vi "config CANcoder.vi"(8 "error in (no error)":errorcluster, 11 "CANcoder init data":T1={"description"="", "Installed?"=FALSE, "CAN ID"=0, "CAN Bus"="", "refnum name"="", "Sensor Direction"=FALSE, "Magnet Offset (Degrees)"=0.0, "gear ratio"=1.0} {"gear ratio" format="%_5f"}) -> (0 "error out":errorcluster)   [LabVIEW 2023]
uses:
  ctrl defs/ctrl CANcoder.ctl
  <vilib>/Rock Robotics/WPI/ThirdParty/Phoenix-LabVIEW/CANCoder/Controls/CTRE_Phoenix_CANcoder_Configurables.ctl
  <vilib>/Rock Robotics/WPI/ThirdParty/Phoenix-LabVIEW/CANCoder/Controls/CTRE_Phoenix_CANcoder_SensorInitializationStrategy.ctl
  <vilib>/Rock Robotics/WPI/ThirdParty/Phoenix-LabVIEW/CANCoder/Controls/CTRE_Phoenix_CANcoder_AbsoluteSensorRange.ctl
  <vilib>/Rock Robotics/WPI/ThirdParty/Phoenix-LabVIEW/Motor Controller/Controls/CTRE_Phoenix_MotorControl_VelocityMeasurementPeriod.ctl
  <vilib>/Rock Robotics/WPI/ThirdParty/Phoenix-LabVIEW/CANCoder/Controls/CTRE_Phoenix_CANcoder_SensorTimeBase.ctl
  <vilib>/Rock Robotics/WPI/ThirdParty/Phoenix-LabVIEW/CANCoder/Set/CTRE_Phoenix_CANcoder_SetPositionToAbsolute.vi
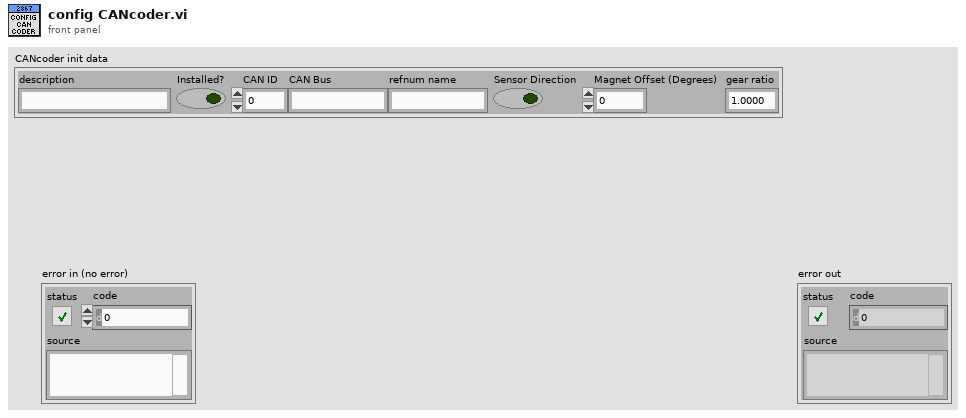
[diagram p1: front panel]
types:
  T1 = typedef "ctrl CANcoder.ctl" = cluster{"description":string, "Installed?":bool, "CAN ID":u8, "CAN Bus":string, "refnum name":string, "Sensor Direction":bool, "Magnet Offset (Degrees)":dbl, "gear ratio":dbl}
  T2 = typedef "CTRE_Phoenix_CANcoder_Configurables.ctl" = cluster{"Sensor Initialization Strategy":T3, "Absolute Sensor Range":T4, "Velocity Measurement Period":T5, "Velocity Measurement Window":i32, "Magnet Offset (Degrees)":dbl, "Sensor Direction":bool, "Sensor Coefficient":dbl, "Unit String":string, "Sensor Time Base":T6}
  T3 = typedef "CTRE_Phoenix_CANcoder_SensorInitializationStrategy.ctl" = enum16{"Boot To Zero", "Boot To Absolute Position"}
  T4 = typedef "CTRE_Phoenix_CANcoder_AbsoluteSensorRange.ctl" = enum16{"Unsigned [0 to 360)", "Signed [-180 to +180)"}
  T5 = typedef "CTRE_Phoenix_MotorControl_VelocityMeasurementPeriod.ctl" = u16
  T6 = typedef "CTRE_Phoenix_CANcoder_SensorTimeBase.ctl" = enum16{"Per100Ms_Legacy", "PerSecond", "PerMinute"}
  T7 = typedef "CTRE_Phoenix_CANcoder_DeviceRef.ctl" = cluster{"DeviceStatus":errorcluster, "Device Number":u8, "Handle":u64, "UsageFrame":u32, "Library Path":path}
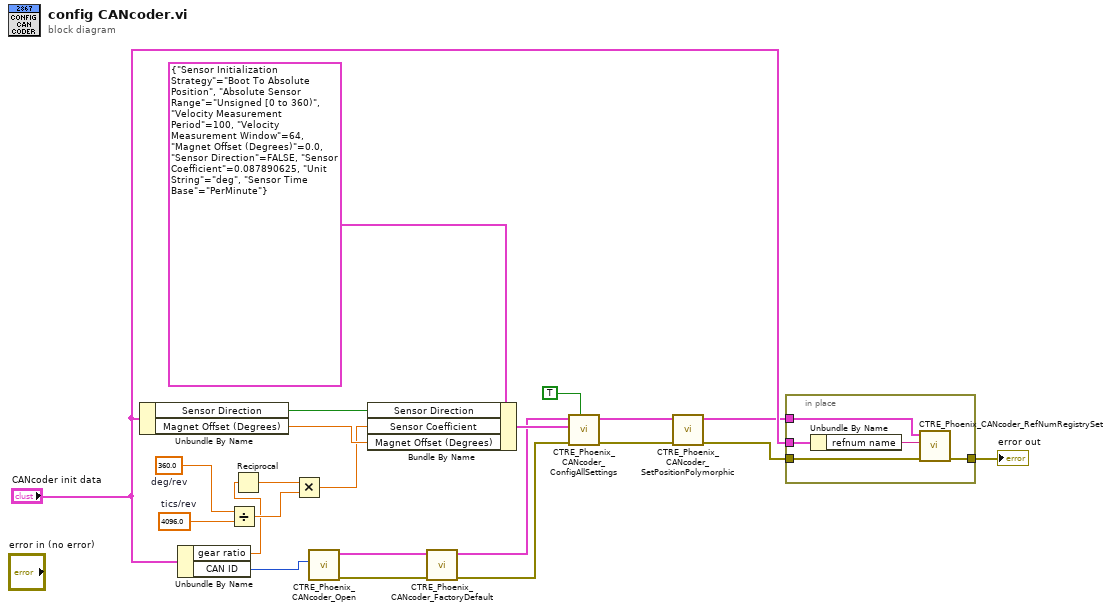
[diagram p0: block diagram]
diagram:
  w4 = 4096.0  # tics/rev
  w5 = 360.0  # deg/rev
  n1 = Unbundle By Name("CANcoder init data") -> ("Sensor Direction"=w14:bool, "Magnet Offset (Degrees)"=w13:dbl)
  n2 = Unbundle By Name("CANcoder init data") -> ("gear ratio"=w2:dbl, "CAN ID"=w21:u8)
  n3 = Divide(x=w5, y=w4) -> (x/y=w3:dbl)
  n4 = Reciprocal(x=w2) -> (1/x=w6:dbl)
  n5 = Multiply(x=w6, y=w3) -> (x*y=w1:dbl)
  n6 = call <vilib>:"CTRE_Phoenix_CANcoder_Open.vi"("Device Number"=w21) -> ("error out"=w20:errorcluster, "CTRE_CANcoder_DeviceRef"=w22:T7)  [unwired: 9 in]
  n7 = Bundle By Name(cluster=T2 {"Sensor Initialization Strategy"=enum."Boot To Absolute Position", "Absolute Sensor Range"=enum."Unsigned [0 to 360)", "Velocity Measurement Period"=100, "Velocity Measurement Window"=64, "Magnet Offset (Degrees)"=0.0, "Sensor Direction"=FALSE, "Sensor Coefficient"=0.087890625, "Unit String"="deg", "Sensor Time Base"=enum."PerMinute"} ("CANcoder Configurables"), "Sensor Direction"=w14, "Sensor Coefficient"=w1, "Magnet Offset (Degrees)"=w13) -> (w15:T2)
  n8 = call <vilib>:"CTRE_Phoenix_CANcoder_FactoryDefault.vi"("error in"=w20, "CTRE_CANcoder_DeviceRef"=w22) -> ("error out"=w11:errorcluster, "CTRE_CANcoder_DeviceRef"=w12:T7)  [unwired: 8 in]
  n9 = call <vilib>:"CTRE_Phoenix_CANcoder_ConfigAllSettings.vi"("Force Write"=TRUE, "error in (no error)"=w11, "CANcoder Configurables"=w15, "CTRE_CANcoder_DeviceRef"=w12) -> ("error out"=w9:errorcluster, "CTRE_CANcoder_DeviceRef"=w10:T7)  [unwired: 6 in]
  n10 = call-poly <vilib>:"CTRE_Phoenix_CANcoder_SetPositionPolymorphic.vi"("error in (no error)"=w9, "CTRE_CANcoder_DeviceRef"=w10) -> ("error out"=w7:errorcluster, "CTRE_CANcoder_DeviceRef"=w8:T7)  [unwired: 8 in]
  n11 = in-place {
    in-place-border: [w26] -> w19
    in-place-border: "CANcoder init data" -> [w25]
    in-place-border: w8 -> [w24]
    in-place-border: w7 -> [w23]
    n12 = Unbundle By Name(w25) -> ("refnum name"=w27:string)
    n13 = call <vilib>:"CTRE_Phoenix_CANcoder_RefNumRegistrySet.vi"("error in (no error)"=w23, "refnum name"=w27, "CTRE_CANcoder_DeviceRef"=w24) -> ("error out"=w26:errorcluster)  [unwired: 7 in, 1 out]
  }
  "error out" <- w19
